vi "close all.vi"(8 "error in (no error)":errorcluster, 11 "5785_3.2GHz_one channel in":refnum<class "5785_3.2GHz_one channel.lvclass">) -> (0 "error out":errorcluster, 3 "5785_3.2GHz_one channel out":refnum<class "5785_3.2GHz_one channel.lvclass">)   [LabVIEW 2021, in "5785_3.2GHz_one channel.lvclass"]
uses:
  5785_3.2GHz_one channel.lvclass
  5785_3.2GHz_one channel.lvclass/5785_3.2GHz_one channel.ctl
  <vilib>/rvi/interface/nirviCloseFPGA/nirviCloseFPGA.xnode
  <vilib>/FPGAPlugInAG/Dynamic/niLvFpga_Close_Dynamic.vi
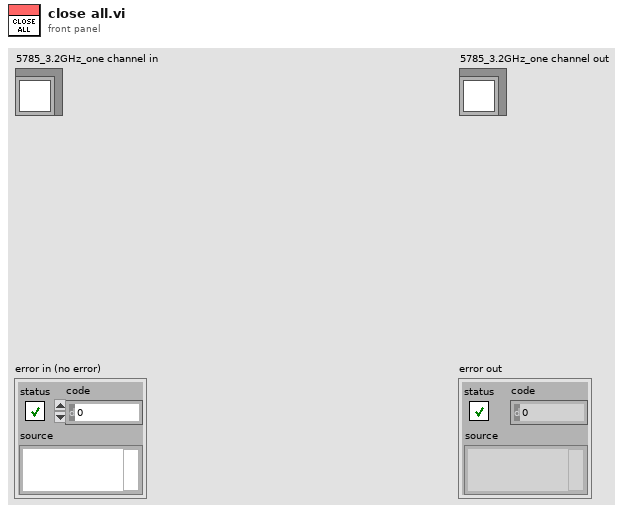
[diagram p1: front panel]
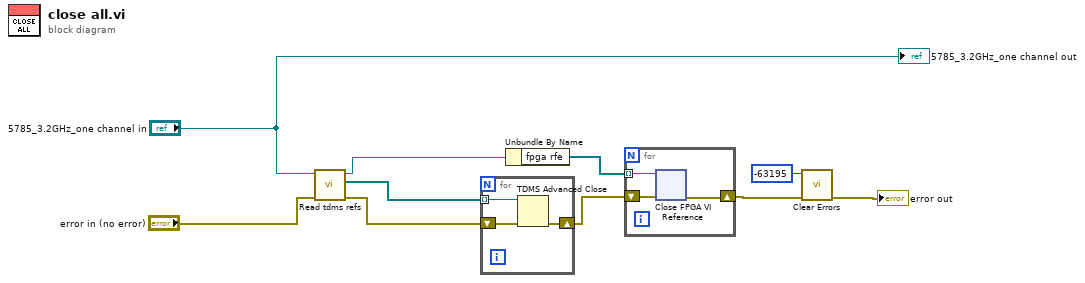
[diagram p0: block diagram]
diagram:
  n1 = call-dynamic "Read tdms refs.vi"("error in (no error)"="error in (no error)", "device_type in"="5785_3.2GHz_one channel in") -> ("error out"=w2:errorcluster, "tdms refs"=w4:refnum<k34>[], "device_type out"=w1:refnum<class "5785_3.2GHz_one channel.lvclass">)  [unwired: 7 in]
  n2 = for {
    shift-right: [w12] -> w10
    shift-left: w2 -> [w13]
    tunnel: w4 -> [w11] mode=indexing
    n3 = TDMS Advanced Close(8:w13, 11:w11) -> (0:w12:errorcluster)  [unwired: 2 in, 1 out]
  }
  n4 = Unbundle By Name(w1) -> ("fpga rfe"=w9:refnum<k20>[])
  n5 = for {
    shift-right: [w15] -> w7
    shift-left: w10 -> [w16]
    tunnel: w9 -> [w14] mode=indexing
    n6 = xnode "Close FPGA VI Reference"("FPGA VI Reference In"=w14, "error in"=w16) -> ("error out"=w15:errorcluster)
  }
  n7 = call <vilib>:"Clear Errors.vi"("error in (no error)"=w7, "specific error code to clear (0: all)"=-63195) -> ("error out"=→"error out":errorcluster)  [unwired: 4 in, 1 out]
  "5785_3.2GHz_one channel out" <- "5785_3.2GHz_one channel in"
